vi "Close_Client.vi"   [LabVIEW 2020]
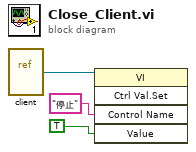
[diagram p0: block diagram]
diagram:
  n1 = vi-ref "client.vi"() -> (w3:refnum<vi>)
  n2 = invoke class="VI" method="Ctrl Val.Set"(reference=w3, "Control Name"="停止" ("控件名"), "Value"=TRUE) -> ()  [unwired: 2 in, 5 out]
